vi "CuLab_Power_Spec_CSG.vi"(7 "window":u16(ring) items=["None "=0, "Hanning"=1, "Hamming"=2, "Blackman-Harris"=3, "Exact Blackman"=4, "Blackman"=5, "Flat Top"=6, "4 Term B-Harris "=7, "7 Term B-Harris"=8, "Low Sidelobe"=9, "Blackman Nuttall"=11], 8 "error in (no error)":errorcluster, 11 "T1D_CSG in":refnum<class "T1D_CSG.lvclass">) -> (0 "error out":errorcluster, 3 "log(x)":refnum<class "T1D_SGL.lvclass">)   [LabVIEW 2020]
uses:
  <vilib>/Ngene/CuLab - GPU Accelerated Toolkit/Toolkit/Low_Level/Tensor_Classes/T_Children/T1D/T1D_Children/T1D_CSG/T1D_CSG.lvclass
  <vilib>/Ngene/CuLab - GPU Accelerated Toolkit/Toolkit/Low_Level/Tensor_Classes/T_Children/T1D/T1D_Children/T1D_SGL/T1D_SGL.lvclass
  <vilib>/Ngene/CuLab - GPU Accelerated Toolkit/Toolkit/API/Signal Processing/Spectral/Power Spectrum/CU_Power_Spectrum_T1D_CSG.vi
  <vilib>/Ngene/CuLab - GPU Accelerated Toolkit/Toolkit/API/Numeric/Add/T1D/CU_AddC_T1D_SGL.vi
  <vilib>/Ngene/CuLab - GPU Accelerated Toolkit/Toolkit/API/Elementary/Exponential/Logarithm Base 10/T1D/CU_Logarithm_Base_10_T1D_SGL.vi
  <vilib>/Ngene/CuLab - GPU Accelerated Toolkit/Toolkit/API/Numeric/Multiply/T1D/CU_MultiplyC_T1D_SGL.vi
  <vilib>/Ngene/CuLab - GPU Accelerated Toolkit/Toolkit/CuLab.lvlib
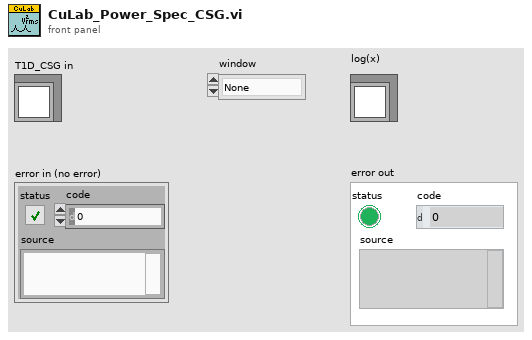
[diagram p1: front panel]
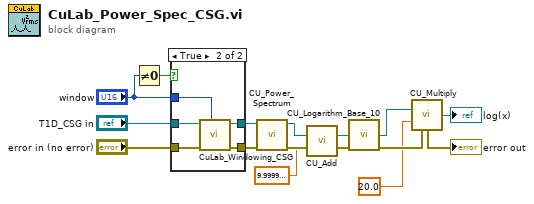
[diagram p0: block diagram]
diagram:
  n1 = Not Equal To 0?(x="window") -> (x != 0?=w3:bool)
  n2 = case shown="True" w3 {
    tunnel: "T1D_CSG in" -> [w17 w22]
    tunnel: [w17 w21] -> w7
    tunnel: "error in (no error)" -> [w16 w20]
    tunnel: [w16 w19] -> w5
    tunnel: "window" -> [_ w18]
    frame False {
    }
    frame True {
      n3 = call "CuLab_Windowing_CSG.vi"("window"=w18, "error in (no error)"=w20, "T1D_CSG in"=w22) -> ("error out"=w19:errorcluster, "T1D_CSG out"=w21:refnum<class "T1D_CSG.lvclass">)  [unwired: 7 in]
    }
  }
  n4 = call-poly <vilib>:"CU_Power_Spectrum.vi"("error in"=w5, "X"=w7) -> ("error out"=w14:errorcluster, "Power Spectrum"=w15:refnum<class "T1D_SGL.lvclass">)  [unwired: 8 in]
  n5 = call-poly <vilib>:"CU_Add.vi"("x"=w15, "y"=sgl 1e-20 ("dt")) -> ("Dest out"=w2:refnum<class "T1D_SGL.lvclass">)  [unwired: 12 in, 1 out]
  n6 = call-poly <vilib>:"CU_Logarithm_Base_10.vi"("x"=w2, "error in (no error)"=w14) -> ("log(x)"=w11:refnum<class "T1D_SGL.lvclass">, "error out"=w12:errorcluster)  [unwired: 12 in]
  n7 = call-poly <vilib>:"CU_Multiply.vi"("x"=w11, "y"=sgl 20.0 ("dt"), "error in (no error)"=w12) -> ("Dest out"=→"log(x)":refnum<class "T1D_SGL.lvclass">, "error out"=→"error out":errorcluster)  [unwired: 11 in]
